vi "TestManyUniqueVariables.vi"() -> ()   [LabVIEW 2018]
uses:
  SendStuff/SlowLogger.lvclass
  SendStuff/SlowLogger.lvclass/SlowLogger.ctl
  b09138e5-eacc-4108-9e9b-99da23817eb2.vi
  b09138e5-eacc-4108-9e9b-99da23817eb2.vi/10ae715b-250f-4b7d-8cc6-608f33e99788.vi
  SendStuff/SlowLogger_LogGEMBANK.vi
  feGEM DataPacker.lvlib
panel:
  out "timed out?":bool
  in  "Number of arrays":i32
  out "Logging Error out":errorcluster
  in  "Max Log Speed [Delta Time] (seconds)":dbl=10.0
  in  "Double array":dbl[](array[numeric])=[0.1, 0.2, 0.3, 0.4, 0.5, 0.6, 0.7, 0.8, 0.9, 1.0]
  in  "stop":bool
  in  "MIDAS Sever Port":u16=12345
  in  "MIDAS Server":string="my_midas_server.domain"
  out "DataPacker Error out":errorcluster
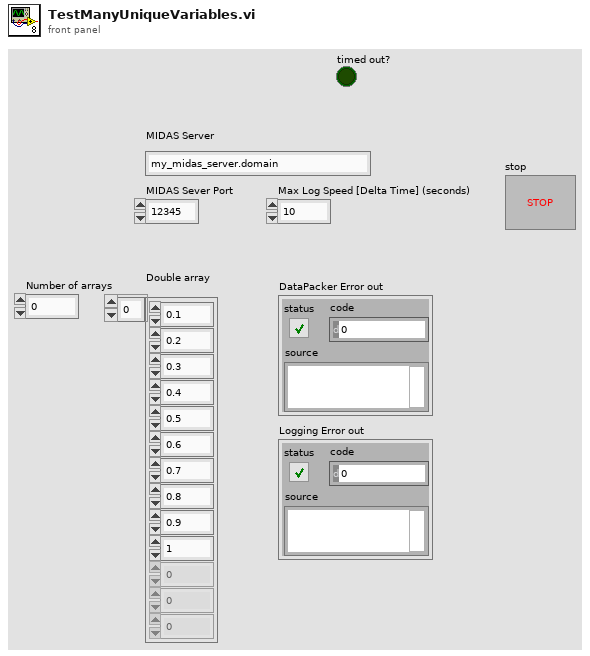
[diagram p1: front panel]
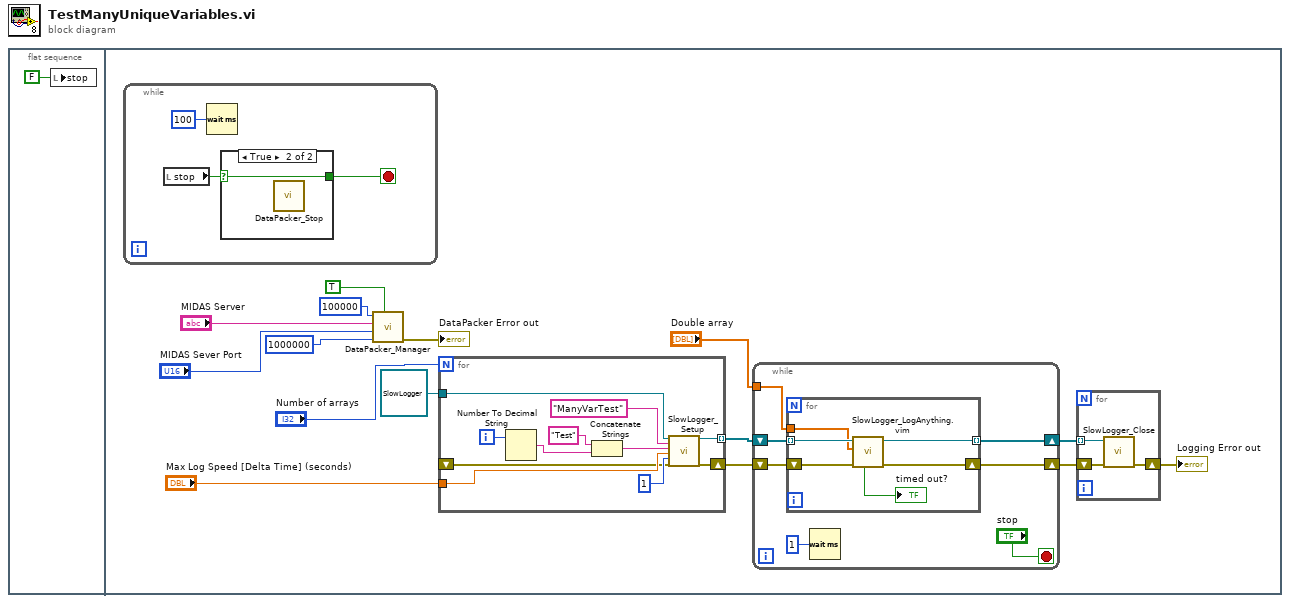
[diagram p0: block diagram]
diagram:
  n1 = flat-sequence {
    frame #0 {
      n2 = local write "stop"(FALSE ("stop")) -> ()
    }
    frame #1 {
      n3 = while {
        stop <- w32 stop-if-true
        n4 = local read "stop"() -> (w31:bool)
        n5 = Wait (ms)(milliseconds to wait=u32 100) -> ()  [unwired: 1 out]
        n6 = case shown="True" w31 {
          selector: w31 -> [w34 w35]
          tunnel: [w34 w35] -> w32
          frame False {
          }
          frame True {
            n7 = call "DataPacker_Stop.vi"() -> ()  [unwired: 12 in]
          }
        }
      }
      n8 = call "DataPacker_Manager.vi"("Request Debug Mode"=TRUE, "max queue size (-1=unlimited)"=1000000, "MIDAS Sever Port"="MIDAS Sever Port", "MIDAS Server"="MIDAS Server", "Override Max Event size (Data rate bytes/s). Use MIDAS Default = 0"=u32 100000 ("Override Max Event size (Data rate kb/s). Use MIDAS Default = 0")) -> ("error out"=→"DataPacker Error out":errorcluster)  [unwired: 6 in]
      n9 = for {
        N: "Number of arrays" -> [_]
        tunnel: refnum<class "SlowLogger.lvclass"> refnum ("feGEM DataPacker.lvlib:SlowLogger.lvclass") -> [w30]
        tunnel: [w29] -> w11 mode=indexing
        tunnel: "Max Log Speed [Delta Time] (seconds)" -> [w22]
        shift-right: [w21] -> w6
        shift-left: _ -> [w20]
        i -> [w26]
        n10 = Number To Decimal String(number=w26) -> (decimal integer string=w25:string)  [unwired: 1 in]
        n11 = Concatenate Strings("Test" ("string"), w25) -> (w24:string)
        n12 = call "SlowLogger_Setup.vi"("SlowLogger in"=w30, "Category"="ManyVarTest", "Variable Name"=w24, "Max Log Speed [Delta Time] (seconds)"=w22, "Period to update history plots (seconds)\nUnset (65535) = Use MIDAS default in ODB\n0 = Record but do not put in histories"=u16 1 ("Period to update history plots (seconds)\nUnset (65535) = Use MIDAS default in ODB\n0 = Record but do not put in histories"), "error in (no error)"=w20) -> ("SlowLogger out"=w29:refnum<class "SlowLogger.lvclass">, "error out"=w21:errorcluster)  [unwired: 12 in]
      }
      n13 = while {
        tunnel: "Double array" -> [w38]
        shift-right: [w39] -> w9
        shift-left: w11 -> [w40]
        shift-right: [w36] -> w5
        shift-left: w6 -> [w37]
        stop <- "stop" stop-if-true
        n14 = for {
          tunnel: w40 -> [w48] mode=indexing
          tunnel: [w46] -> w39 mode=indexing
          tunnel: w38 -> [w47]
          shift-right: [w44] -> w36
          shift-left: w37 -> [w45]
          n15 = call "SlowLogger_LogAnything.vim"("error in"=w45, "Array"=w47, "SlowLogger in"=w48) -> ("error out"=w44:errorcluster, "SlowLogger out"=w46:refnum<class "SlowLogger.lvclass">, "timed out?"=→"timed out?":bool)  [unwired: 4 in, 2 out]
        }
        n16 = Wait (ms)(milliseconds to wait=u32 1) -> ()  [unwired: 1 out]
      }
      n17 = for {
        tunnel: w9 -> [w19] mode=indexing
        shift-right: [w17] -> w4
        shift-left: w5 -> [w18]
        n18 = call "SlowLogger_Close.vi"("error in (no error)"=w18, "SlowLogger in"=w19) -> ("error out"=w17:errorcluster)  [unwired: 9 in]
      }
      "Logging Error out" <- w4
    }
  }
